vi "Write.vi"(8 "error in (no error)":errorcluster, 10 "write buffer":string, 11 "Serial in":refnum<class "Mock Serial.lvclass">) -> (0 "error out":errorcluster, 2 "return count":u32, 3 "Serial out":refnum<class "Mock Serial.lvclass">)   [LabVIEW 2020, in "Mock Serial.lvclass"]
uses:
  Mock Serial.lvclass
  C:/git/astemes-lmock/source/Framework/Mock/LMock Mock.lvclass
  Framework/Mock/LMock Mock.lvclass
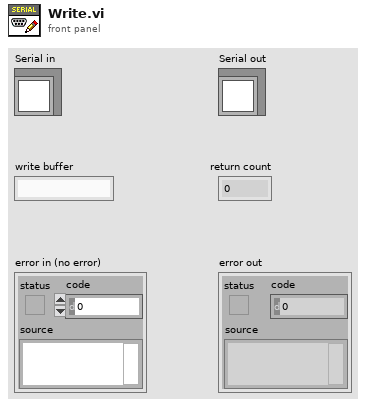
[diagram p1: front panel]
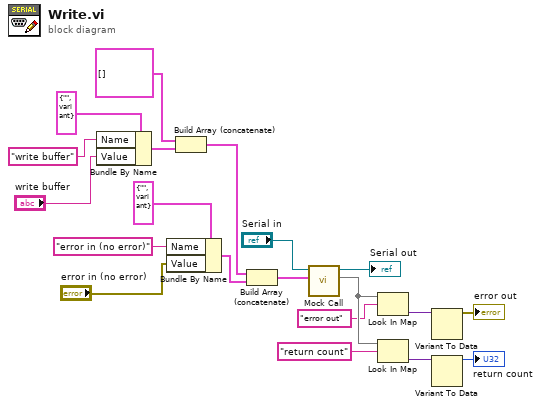
[diagram p0: block diagram]
diagram:
  n1 = Bundle By Name(cluster=cluster{"Name":string, "Value":variant} {"Name"="", "Value"=variant} ("element"), "Name"="write buffer", "Value"="write buffer") -> (w3:cluster{"Name":string, "Value":variant})
  n2 = Bundle By Name(cluster=cluster{"Name":string, "Value":variant} {"Name"="", "Value"=variant} ("element"), "Name"="error in (no error)", "Value"="error in (no error)") -> (w1:cluster{"Name":string, "Value":variant})
  n3 = Build Array (concatenate)(cluster{"Name":string, "Value":variant}[] [] ("Control Values"), w3) -> (w15:cluster{"Name":string, "Value":variant}[])
  n4 = Build Array (concatenate)(w15, w1) -> (w17:cluster{"Name":string, "Value":variant}[])
  n5 = call "Mock Call.vi"("Control Values"=w17, "Mock In"="Serial in") -> ("Return Values"=w12:map{string, variant}, "Mock Out"=→"Serial out":refnum<class "Mock Serial.lvclass">)  [unwired: 8 in]
  n6 = Look In Map(map=w12, key="error out") -> (value=w10:variant)  [unwired: 1 in, 1 out]
  n7 = Look In Map(map=w12, key="return count") -> (value=w7:variant)  [unwired: 1 in, 1 out]
  n8 = Variant To Data(Variant=w10) -> (data=→"error out":errorcluster)  [unwired: 2 in, 1 out]
  n9 = Variant To Data(Variant=w7) -> (data=→"return count":u32)  [unwired: 2 in, 1 out]
